vi "meth.PushVarArray.vi"(0 "class.GLue in":refnum<class "class.GLue.lvclass">, 7 "VarArray":variant, 11 "error in (no error)":errorcluster) -> (4 "class.GLue out":refnum<class "class.GLue.lvclass">, 8 "Pushed?":bool=TRUE, 15 "error out":errorcluster)   [LabVIEW 2014, in "GLue.lvlib" / "class.GLue.lvclass"]
uses:
  class.GLue.lvclass
  class.GLue.lvclass/class.GLue.ctl
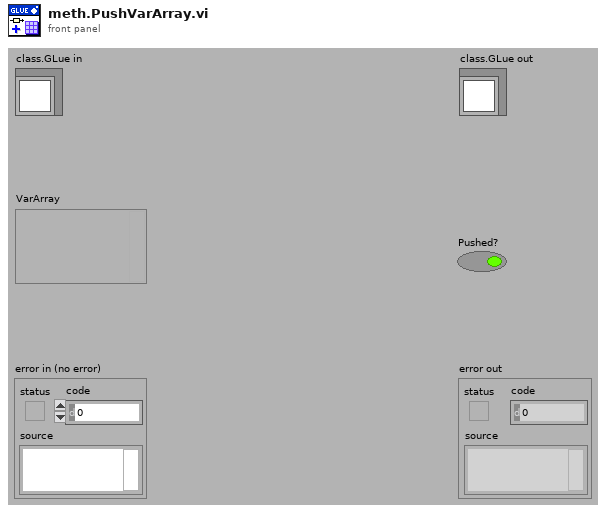
[diagram p1: front panel]
types:
  T1 = enum8{"<Null>", "I8", "I16", "I32", "I64", "U8", "U16", "U32", "U64", "SGL", "DBL", "EXT", "CSG", "CDB", "CXT", "0x0F", "0x10", "0x11", "0x12", "0x13", "0x14", "Enum U8", "Enum U16", "Enum U32", "Enum U64", "SGL PQ", "DBL PQ", "EXT PQ", "CSG PQ", "CDB PQ", "CXT PQ", "0x1F", "0x20", "Boolean", "0x22", "0x23", "0x24", "0x25", "0x26", "0x27", "0x28", "0x29", "0x2A", "0x2B", "0x2C", "0x2D", "0x2E", "0x2F", "String", "0x31", "Path", "Pict", "0x34", "0x35", "0x36", "DAQ", "0x38", "0x39", "0x3A", "0x3B", "0x3C", "0x3D", "0x3E", "0x3F", "Array", "0x41", "0x42", "0x43", "0x44", "0x45", "0x46", "0x47", "0x48", "0x49", "0x4A", "0x4B", "0x4C", "0x4D", "0x4E", "0x4F", "Cluster", "0x51", "0x52", "Variant", "Waveform", "0x55", "0x56", "0x57", "0x58", "0x59", "0x5A", "0x5B", "0x5C", "0x5D", "0x5E", "0x5F", "0x60", "0x61", "0x62", "0x63", "0x64", "0x65", "0x66", "0x67", "0x68", "0x69", "0x6A", "0x6B", "0x6C", "0x6D", "0x6E", "0x6F", "Refnum"}
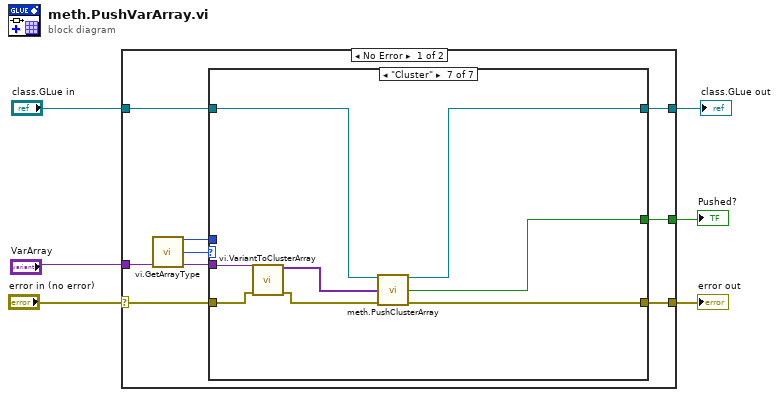
[diagram p0: block diagram]
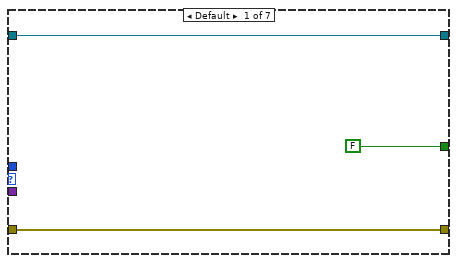
[diagram p2: hidden frame]
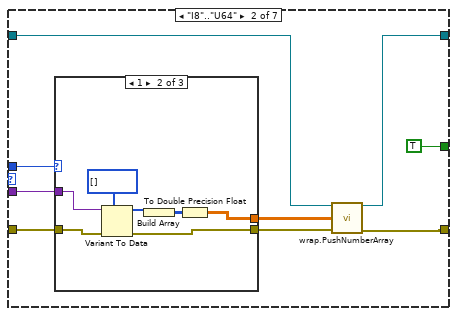
[diagram p3: hidden frame]
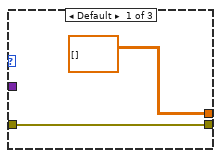
[diagram p4: hidden frame]
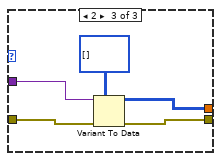
[diagram p5: hidden frame]
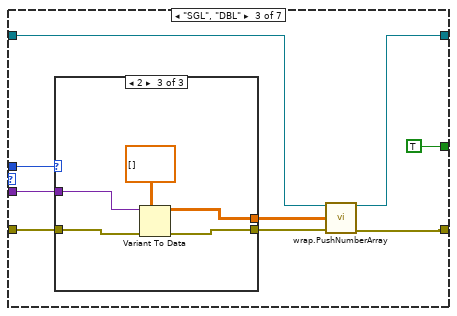
[diagram p6: hidden frame]
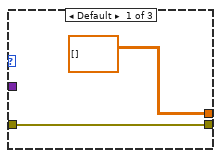
[diagram p7: hidden frame]
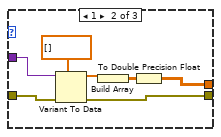
[diagram p8: hidden frame]
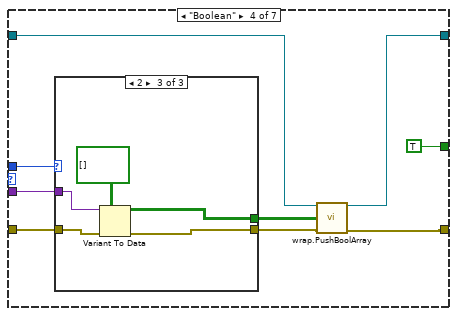
[diagram p9: hidden frame]
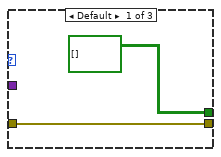
[diagram p10: hidden frame]
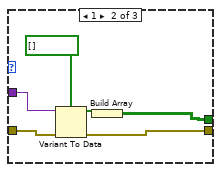
[diagram p11: hidden frame]
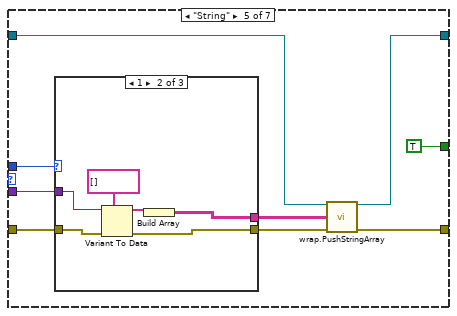
[diagram p12: hidden frame]
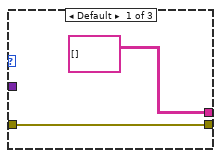
[diagram p13: hidden frame]
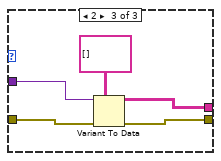
[diagram p14: hidden frame]
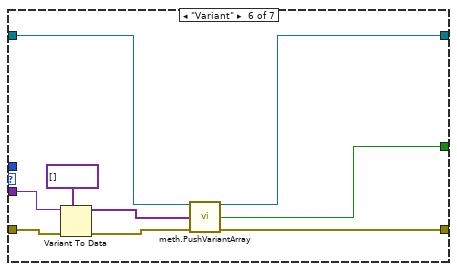
[diagram p15: hidden frame]
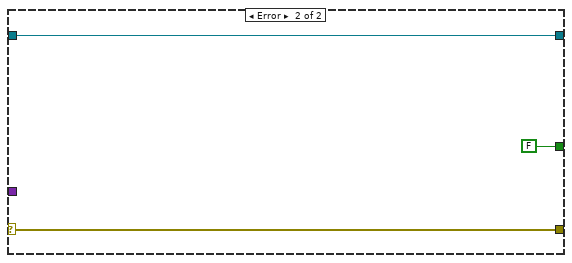
[diagram p16: hidden frame]
diagram:
  n1 = case shown="No Error" "error in (no error)" {
    selector: "error in (no error)" -> [w13 w128]
    tunnel: [w12 w128] -> w5
    tunnel: [w14 w127] -> w3
    tunnel: "class.GLue in" -> [w15 w127]
    tunnel: "VarArray" -> [w11 _]
    tunnel: [w7 FALSE] -> w1
    frame No Error {
      n2 = call "vi.GetArrayType.vi"("VarArray in"=w11) -> ("Dims"=w8:u32, "type"=w10:T1, "VarArray out"=w9:variant)  [unwired: 12 in]
      n3 = case shown="\"Cluster\"" w10 {
        tunnel: w15 -> [w18 w21 w44 w69 w92 w116 w120]
        tunnel: [w18 w20 w43 w68 w91 w115 w119] -> w14
        tunnel: w13 -> [w17 w27 w50 w73 w95 w113 w124]
        tunnel: [w17 w23 w46 w66 w88 w117 w122] -> w12
        tunnel: w9 -> [_ w26 w49 w72 w94 w111 w125]
        tunnel: w8 -> [_ w25 w48 w71 w93 _ _]
        tunnel: [FALSE TRUE TRUE TRUE TRUE w114 w118] -> w7
        frame Default {
        }
        frame "I8".."U64" {
          n4 = case shown="1" w25 {
            tunnel: w27 -> [w29 w36 w41]
            tunnel: [w29 w31 w38] -> w24
            tunnel: w26 -> [_ w35 w40]
            tunnel: [dbl[][] [] w30 w37] -> w22
            frame Default {
            }
            frame 1 {
              n5 = Variant To Data(error in=w36, type=i32[] [], Variant=w35) -> (data=w33:i32[], error out=w31:errorcluster)
              n6 = Build Array(w33) -> (w32:i32[][])
              n7 = To Double Precision Float(number=w32) -> (double precision float=w30:dbl[][])
            }
            frame 2 {
              n8 = Variant To Data(error in=w41, type=i32[][] [], Variant=w40) -> (data=w37:i32[][], error out=w38:errorcluster)
            }
          }
          n9 = call "wrap.PushNumberArray.vi"("class.GLue in"=w21, "FloatArray"=w22, "error in (no error)"=w24) -> ("class.GLue out"=w20:refnum<class "class.GLue.lvclass">, "error out"=w23:errorcluster)  [unwired: 11 in]
        }
        frame "SGL", "DBL" {
          n10 = case shown="2" w48 {
            tunnel: w50 -> [w52 w59 w64]
            tunnel: [w52 w54 w61] -> w47
            tunnel: w49 -> [_ w58 w63]
            tunnel: [dbl[][] [] w53 w60] -> w45
            frame Default {
            }
            frame 1 {
              n11 = Variant To Data(error in=w59, type=dbl[] [], Variant=w58) -> (data=w56:dbl[], error out=w54:errorcluster)
              n12 = Build Array(w56) -> (w55:dbl[][])
              n13 = To Double Precision Float(number=w55) -> (double precision float=w53:dbl[][])
            }
            frame 2 {
              n14 = Variant To Data(error in=w64, type=dbl[][] [], Variant=w63) -> (data=w60:dbl[][], error out=w61:errorcluster)
            }
          }
          n15 = call "wrap.PushNumberArray.vi"("class.GLue in"=w44, "FloatArray"=w45, "error in (no error)"=w47) -> ("class.GLue out"=w43:refnum<class "class.GLue.lvclass">, "error out"=w46:errorcluster)  [unwired: 11 in]
        }
        frame "Boolean" {
          n16 = case shown="2" w71 {
            tunnel: w73 -> [w75 w81 w86]
            tunnel: [w75 w78 w84] -> w67
            tunnel: w72 -> [_ w80 w85]
            tunnel: [bool[][] [] w76 w82] -> w65
            frame Default {
            }
            frame 1 {
              n17 = Variant To Data(error in=w81, type=bool[] [], Variant=w80) -> (data=w79:bool[], error out=w78:errorcluster)
              n18 = Build Array(w79) -> (w76:bool[][])
            }
            frame 2 {
              n19 = Variant To Data(error in=w86, type=bool[][] [], Variant=w85) -> (data=w82:bool[][], error out=w84:errorcluster)
            }
          }
          n20 = call "wrap.PushBoolArray.vi"("class.GLue in"=w69, "BoolArray"=w65, "error in (no error)"=w67) -> ("class.GLue out"=w68:refnum<class "class.GLue.lvclass">, "error out"=w66:errorcluster)  [unwired: 11 in]
        }
        frame "String" {
          n21 = case shown="1" w93 {
            tunnel: w95 -> [w97 w103 w108]
            tunnel: [w97 w99 w105] -> w89
            tunnel: w94 -> [_ w102 w107]
            tunnel: [string[][] [] w98 w104] -> w90
            frame Default {
            }
            frame 1 {
              n22 = Variant To Data(error in=w103, type=string[] [], Variant=w102) -> (data=w100:string[], error out=w99:errorcluster)
              n23 = Build Array(w100) -> (w98:string[][])
            }
            frame 2 {
              n24 = Variant To Data(error in=w108, type=string[][] [], Variant=w107) -> (data=w104:string[][], error out=w105:errorcluster)
            }
          }
          n25 = call "wrap.PushStringArray.vi"("class.GLue in"=w92, "StringArray"=w90, "error in (no error)"=w89) -> ("class.GLue out"=w91:refnum<class "class.GLue.lvclass">, "error out"=w88:errorcluster)  [unwired: 11 in]
        }
        frame "Variant" {
          n26 = Variant To Data(error in=w113, type=variant[] [], Variant=w111) -> (data=w109:variant[], error out=w112:errorcluster)
          n27 = call "meth.PushVariantArray.vi"("class.GLue in"=w116, "Array"=w109, "error in"=w112) -> ("class.GLue out"=w115:refnum<class "class.GLue.lvclass">, "Pushed?"=w114:bool, "error out"=w117:errorcluster)  [unwired: 10 in]
        }
        frame "Cluster" {
          n28 = call "vi.VariantToClusterArray.vi"("ClusterArray"=w125, "error in"=w124) -> ("VariantArray"=w121:variant[], "error out"=w123:errorcluster)  [unwired: 12 in]
          n29 = call "meth.PushClusterArray.vi"("class.GLue in"=w120, "Array"=w121, "error in"=w123) -> ("class.GLue out"=w119:refnum<class "class.GLue.lvclass">, "Pushed?"=w118:bool, "error out"=w122:errorcluster)  [unwired: 10 in]
        }
      }
    }
    frame Error {
    }
  }
  "error out" <- w5
  "class.GLue out" <- w3
  "Pushed?" <- w1
